vi "Send Msg Trigger.vi"(8 "error in (no error)":errorcluster, 9 "Trigger Msg (F)":bool, 10 "PVName":string, 11 "PVConnections":refnum<class "PVConnection.lvclass">[](array[class])) -> (0 "error out":errorcluster, 3 "PVConnection out":refnum<class "PVConnection.lvclass">)   [LabVIEW 2016, in "CS++GUIActor.lvlib" / "CS++GUIActor.lvclass"]
doc: "In GUIs this Vi can be used to send values to Set PVs.\nAs input a list of valid PVConnections is expected (in a GUI execute the Connect-SetPVs.vi first). In the following this VI searches for a PV with a given name and sets the PV if the variable was found."
uses:
  CS++GUIActor.lvclass
  Classes/CS++ProcessVariables/PVConnection/PVConnection.lvclass
  Classes/CS++ProcessVariables/PVConnection/PVConnection.lvclass/PVConnection.ctl
  Classes/CS++ProcessVariables/ProcessVariable/PV.lvclass/PV.ctl
  Classes/CS++ProcessVariables/ProcessVariable/PV.lvclass
panel:
  out "Found?":bool
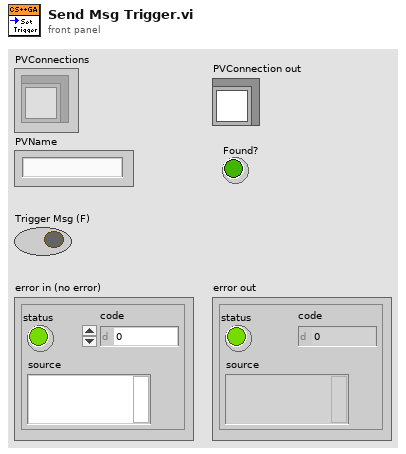
[diagram p1: front panel]
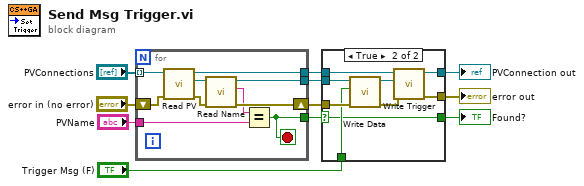
[diagram p0: block diagram]
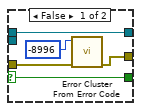
[diagram p2: hidden frame]
diagram:
  n1 = for {
    tunnel: [w21] -> w11
    tunnel: [w17] -> w9
    shift-right: [w16] -> w10
    shift-left: "error in (no error)" -> [w20]
    tunnel: "PVConnections" -> [w19] mode=indexing
    tunnel: "PVName" -> [w13]
    tunnel: [w12] -> w2
    stop <- w12 stop-if-true
    n2 = call "Read PV.vi"("error in (no error)"=w20, "PVConnection in"=w19) -> ("error out"=w15:errorcluster, "PV"=w18:refnum<class "PV.lvclass">, "PVConnection out"=w21:refnum<class "PVConnection.lvclass">)  [unwired: 7 in]
    n3 = call "Read Name.vi"("error in (no error)"=w15, "PV in"=w18) -> ("error out"=w16:errorcluster, "Name"=w14:string, "PV out"=w17:refnum<class "PV.lvclass">)  [unwired: 7 in]
    n4 = Equal?(x=w14, y=w13) -> (x = y?=w12:bool)
  }
  n5 = case shown="True" w2 {
    selector: w2 -> [w25 w32]
    tunnel: w11 -> [w26 w31]
    tunnel: w10 -> [w23 w35]
    tunnel: w9 -> [_ w34]
    tunnel: "Trigger Msg (F)" -> [_ w33]
    tunnel: [w22 w28] -> w6
    tunnel: [w26 w30] -> w5
    tunnel: [w25 w32] -> w1
    frame False {
      n6 = call <vilib>:"Error Cluster From Error Code.vi"("error in (no error)"=w23, "error code (0)"=-8996) -> ("error out"=w22:errorcluster)  [unwired: 7 in]
    }
    frame True {
      n7 = call "Write Data.vi"("error in (no error)"=w35, "Data"=w33, "PV in"=w34) -> ("error out"=w29:errorcluster, "PV out"=w27:refnum<class "PV.lvclass">)  [unwired: 7 in]
      n8 = call "Write Trigger.vi"("error in (no error)"=w29, "PV"=w27, "PVConnection in"=w31) -> ("error out"=w28:errorcluster, "PVConnection out"=w30:refnum<class "PVConnection.lvclass">)  [unwired: 7 in]
    }
  }
  "error out" <- w6
  "PVConnection out" <- w5
  "Found?" <- w1
